vi "FPGAUpdateAO.vi"(2 "AIO cluster":T1, 3 "error in":errorcluster) -> (9 "error out":errorcluster)   [LabVIEW 2019]
uses:
  <vilib>/Utility/error.llb/Error Cluster From Error Code.vi
  <vilib>/rvi/errors/niLvFpgaAdjustHostInterfaceError.vi
  <vilib>/rvi/interface/nirviReadWriteControl/nirviReadWriteControl.xnode
  NiFpgaLv.dll
  <vilib>/rvi/interface/Simulation/niFpgaSimulationCallBeginRW.vi
panel:
  # "AOM"
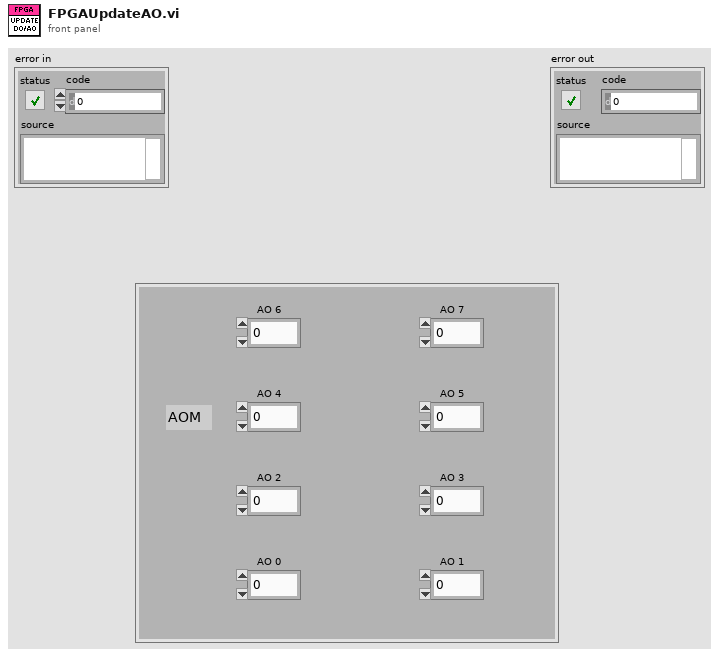
[diagram p1: front panel]
types:
  T1 = cluster{"AO 0":dbl, "AO 1":dbl, "AO 2":dbl, "AO 3":dbl, "AO 4":dbl, "AO 5":dbl, "AO 6":dbl, "AO 7":dbl}
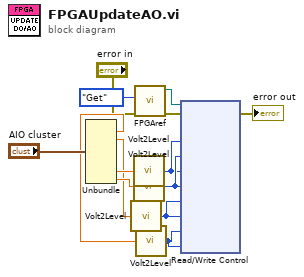
[diagram p0: block diagram]
diagram:
  n1 = Unbundle("AIO cluster") -> ("AO 1"=w5:dbl, "AO 2"=w7:dbl, "AO 6"=w11:dbl, "AO 7"=w10:dbl)  [unwired: 4 out]
  n2 = call "Volt2Level.vi"("voltage /V"=w7) -> ("level"=w6:i16)
  n3 = call "Volt2Level.vi"("voltage /V"=w11) -> ("level"=w8:i16)
  n4 = call "Volt2Level.vi"("voltage /V"=w10) -> ("level"=w9:i16)
  n5 = call "FPGAref.vi"("error in"="error in", "Enum"=enum16{"Set", "Get"}."Get") -> ("error out"=w2:errorcluster, "FPGA VI Reference Out 2"=w13:refnum<k20>)  [unwired: 4 in]
  n6 = call "Volt2Level.vi"("voltage /V"=w5) -> ("level"=w4:i16)
  n7 = xnode "Read/Write Control"("FPGA VI Reference In"=w13, "error in"=w2, "AO6"=w8, "AO7"=w9, "AO6"=w8, "AO7"=w9, "AO2 off"=w6, "AO2 on"=w6, "AO1 off"=w4, "AO1 on"=w4) -> ("error out"=→"error out":errorcluster)  [unwired: 1 in, 1 out]
